vi "averagePoints.vi"(2 "robotPos":cluster{"xPos":dbl, "yPos":dbl, "Theta":dbl}, 3 "Array":T1(array[cluster])) -> (1 "lidarRobotPos":cluster{"xPos":dbl, "yPos":dbl, "Theta":dbl})   [LabVIEW 2016]
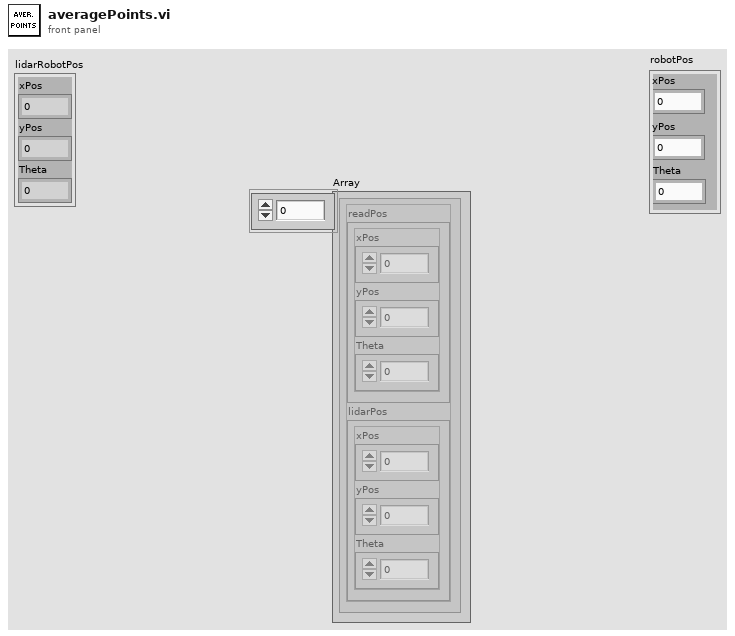
[diagram p1: front panel]
types:
  T1 = cluster{"readPos":cluster{"xPos":dbl, "yPos":dbl, "Theta":dbl}, "lidarPos":cluster{"xPos":dbl, "yPos":dbl, "Theta":dbl}}[]
  T2 = cluster{"readPos":cluster{"xPos":dbl, "yPos":dbl, "Theta":dbl}, "lidarPos":cluster{"xPos":dbl, "yPos":dbl, "Theta":dbl}}
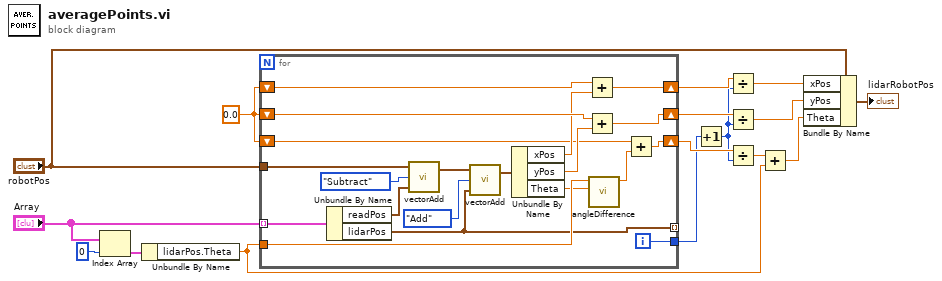
[diagram p0: block diagram]
diagram:
  w7 = 0.0
  n1 = Index Array(array="Array", index=0) -> (element=w5:T2)
  n2 = Unbundle By Name(w5) -> ("lidarPos.Theta"=w3:dbl)
  n3 = for {
    tunnel: [w20] -> _ mode=indexing
    shift-right: [w33] -> w15
    shift-left: w7 -> [w36]
    shift-right: [w34] -> w16
    shift-left: w7 -> [w35]
    shift-right: [w25] -> w12
    shift-left: w7 -> [w27]
    tunnel: [w30] -> w9
    tunnel: w3 -> [w29]
    tunnel: "Array" -> [w24] mode=indexing
    tunnel: "robotPos" -> [w23]
    i -> [w30]
    n4 = Unbundle By Name(w24) -> ("readPos"=w22:cluster{"xPos":dbl, "yPos":dbl, "Theta":dbl}, "lidarPos"=w20:cluster{"xPos":dbl, "yPos":dbl, "Theta":dbl})
    n5 = call "vectorAdd.vi"("b"=w22, "operation"=enum16{"Subtract", "Add"}."Subtract", "a"=w23) -> ("a +/- b"=w21:cluster{"xPos":dbl, "yPos":dbl, "Theta":dbl})  [unwired: 1 in]
    n6 = call "vectorAdd.vi"("b"=w20, "operation"=enum16{"Subtract", "Add"}."Add", "a"=w21) -> ("a +/- b"=w19:cluster{"xPos":dbl, "yPos":dbl, "Theta":dbl})  [unwired: 1 in]
    n7 = Unbundle By Name(w19) -> ("xPos"=w32:dbl, "yPos"=w31:dbl, "Theta"=w28:dbl)
    n8 = Add(x=w36, y=w32) -> (x+y=w33:dbl)
    n9 = Add(x=w35, y=w31) -> (x+y=w34:dbl)
    n10 = call "angleDifference.vi"("theta B"=w28, "theta A"=w29) -> ("delta theta"=w26:dbl)  [unwired: 9 in]
    n11 = Add(x=w27, y=w26) -> (x+y=w25:dbl)
  }
  n12 = Increment(x=w9) -> (x+1=w8:i32)
  n13 = Divide(x=w15, y=w8) -> (x/y=w14:dbl)
  n14 = Divide(x=w16, y=w8) -> (x/y=w13:dbl)
  n15 = Divide(x=w12, y=w8) -> (x/y=w11:dbl)
  n16 = Add(x=w11, y=w3) -> (x+y=w10:dbl)
  n17 = Bundle By Name(cluster="robotPos", "xPos"=w14, "yPos"=w13, "Theta"=w10) -> (→"lidarRobotPos":cluster{"xPos":dbl, "yPos":dbl, "Theta":dbl})
